vi "AH 2550 Single Measurement.vi"() -> ()   [LabVIEW 2016]
doc: "This example shows how to configure the bridge, take a single capacitance measurement, read the results from the bridge, and parse the measurement results."
uses:
  Andeen-Hagerling 2550.lvlib
panel:
  out "Error Code":i32
  out "Sample Switch":i32
  out "Frequency":dbl
  out "Units Display":i32(ring)=1 items=["nanosiemens"=1, "dissipation factor"=2, "kilohms"=3, "gigohms"=4, "loss vector (jpF)"=5]
  out "Applied Voltage":dbl format="%#_6f"
  out "Loss":dbl
  out "Capacitance":dbl format="%#_10f"
  in  "Units":i32(ring)=1 items=["nanosiemens"=1, "dissipation factor"=2, "kilohms"=3, "gigohms"=4, "loss vector (jpF)"=5]
  in  "Maximum Voltage":dbl=15.0 min=0.0003 max=15.0 step=1.0 format="%#.6f"
  in  "Average Exponent":u16=4 max=15
  in  "VISA resource name":refnum<visa-resource-name>
  in  "Serial Configuration":T1={"Baud Rate"=9600, "Parity"=0, "Data Bits"=8, "Stop Bits"=10} {"Stop Bits" items=["1.0"=10, "1.5"=15, "2.0"=20]; "Data Bits" items=["7"=7, "8"=8]; "Parity" items=["None", "Odd", "Even", "Mark", "Space"]; "Baud Rate" items=["300"=300, "600"=600, "1200"=1200, "2400"=2400, "4800"=4800, "9600"=9600, "19200"=19200]}
  # "AH 2550A ULTRA-PRECISION 1kHz CAPACITANCE BRIDGE"
  # "Single Measurement"
  # "Measurement Results"
  # "Measurement Parameters"
  # "picoFarads"
  # "V"
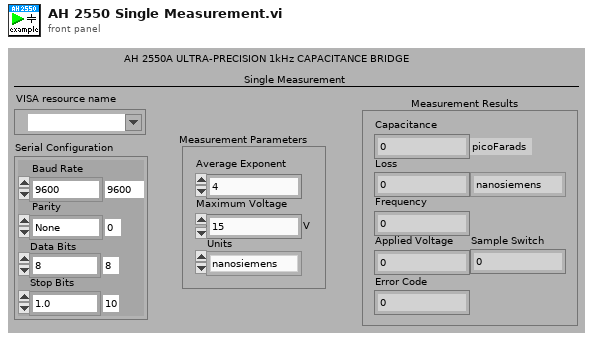
[diagram p1: front panel]
types:
  T1 = cluster{"Baud Rate":u32, "Parity":u16, "Data Bits":u16, "Stop Bits":u16}
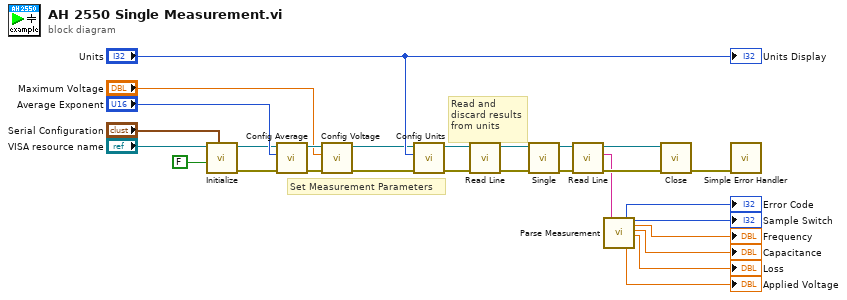
[diagram p0: block diagram]
diagram:
  # "Set Measurement Parameters"
  # "Read and\ndiscard results\nfrom units"
  n1 = call "Initialize.vi"("Serial Configuration"="Serial Configuration", "Reset (True)"=FALSE, "VISA resource name"="VISA resource name") -> ("error out"=w9:errorcluster, "VISA resource name out"=w10:refnum<visa-resource-name>)  [unwired: 7 in]
  n2 = call "Config Average.vi"("error in"=w9, "Average Exponent (4)"="Average Exponent", "VISA resource name"=w10) -> ("error out"=w25:errorcluster, "VISA resource name out"=w26:refnum<visa-resource-name>)  [unwired: 7 in]
  n3 = call "Config Voltage.vi"("error in"=w25, "Voltage (15 V)"="Maximum Voltage", "VISA resource name"=w26) -> ("error out"=w3:errorcluster, "VISA resource name out"=w4:refnum<visa-resource-name>)  [unwired: 7 in]
  n4 = call "Config Units.vi"("error in"=w3, "Units (nS)"="Units", "VISA resource name"=w4) -> ("error out"=w21:errorcluster, "VISA resource name out"=w22:refnum<visa-resource-name>)  [unwired: 7 in]
  n5 = call "Read Line.vi"("error in"=w21, "VISA resource name"=w22) -> ("error out"=w19:errorcluster, "VISA resource name out"=w20:refnum<visa-resource-name>)  [unwired: 5 in, 3 out]
  n6 = call "Single.vi"("error in"=w19, "VISA resource name"=w20) -> ("error out"=w17:errorcluster, "VISA resource name out"=w18:refnum<visa-resource-name>)  [unwired: 8 in]
  n7 = call "Read Line.vi"("error in"=w17, "VISA resource name"=w18) -> ("error out"=w15:errorcluster, "Message"=w14:string, "VISA resource name out"=w16:refnum<visa-resource-name>)  [unwired: 5 in, 2 out]
  n8 = call "Parse Measurement.vi"("Measurement Line"=w14) -> ("Error Code"=→"Error Code":i32, "Voltage"=→"Applied Voltage":dbl, "Sample"=→"Sample Switch":i32, "Frequency"=→"Frequency":dbl, "Capacitance"=→"Capacitance":dbl, "Loss"=→"Loss":dbl)  [unwired: 10 in, 3 out]
  n9 = call "Close.vi"("error in (no error)"=w15, "VISA resource name"=w16) -> ("error out"=w5:errorcluster)  [unwired: 9 in]
  n10 = call <vilib>:"Simple Error Handler.vi"("error in (no error)"=w5) -> ()  [unwired: 4 in, 5 out]
  "Units Display" <- "Units"
